vi "SearchUser.vi"(8 "User":string caption="User Name:", 11 "UserLibFile":path) -> (0 "Group":i32, 1 "Pwd":string, 2 "Index":i32, 3 "Exist?":bool)   [LabVIEW 2020]
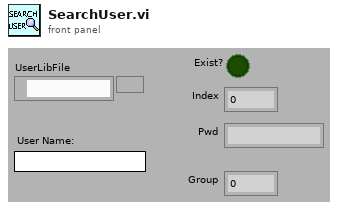
[diagram p1: front panel]
types:
  T1 = enum16{"open", "replace", "create", "open or create", "replace or create", "replace or create with confirmation"}
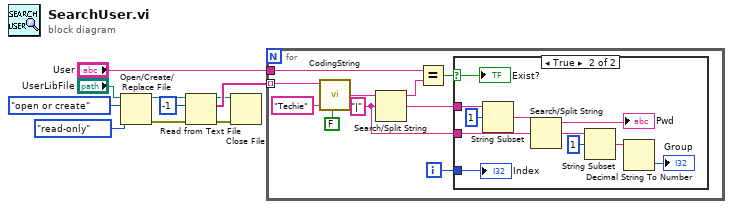
[diagram p0: block diagram]
diagram:
  n1 = Open/Create/Replace File(file path (use dialog)="UserLibFile", operation (0:open)=T1."open or create", access (0:read/write)=enum16{"read/write", "read-only", "write-only"}."read-only") -> (refnum out=w7:refnum<file>, error out=w8:errorcluster)  [unwired: 1 in, 3 out]
  n2 = Read from Text File(file (use dialog)=w7, count=-1, error in=w8) -> (refnum out=w5:refnum<file>, text=w10:string[], error out=w6:errorcluster)  [unwired: 2 out]
  n3 = Close File(refnum=w5, error in=w6) -> ()  [unwired: 2 out]
  n4 = for {
    tunnel: w10 -> [w18] mode=indexing
    tunnel: "User" -> [w11]
    i -> [w15]
    w12 = "|" ("search string/char (-)")
    n5 = call "CodingString.vi"("InputStr"=w18, "key"="Techie", "Coding(T)?"=FALSE) -> ("Output"=w14:string)  [unwired: 1 in, 1 out]
    n6 = Search/Split String(string=w14, search string/char (-)=w12) -> (substring before match=w19:string, match + rest of string=w13:string)  [unwired: 2 out]
    n7 = Equal?(x=w11, y=w19) -> (x = y?=w20:bool)
    n8 = case shown="True" w20 {
      selector: w20 -> [_ w31]
      tunnel: w15 -> [_ w30]
      tunnel: w13 -> [_ w23]
      tunnel: w12 -> [_ w22]
      frame False {
      }
      frame True {
        n9 = String Subset(string=w23, offset (0)=1) -> (substring=w25:string)  [unwired: 1 out]
        n10 = Search/Split String(string=w25, search string/char (-)=w22) -> (substring before match=→"Pwd":string, match + rest of string=w28:string)  [unwired: 2 out]
        n11 = String Subset(string=w28, offset (0)=1) -> (substring=w29:string)  [unwired: 1 out]
        n12 = Decimal String To Number(string=w29) -> (number=→"Group":i32)  [unwired: 3 out]
        "Exist?" <- w31
        "Index" <- w30
      }
    }
  }
